vi "identify region.vi"(3 "index":u8=1, 4 "points":cluster{"x":i16, "y":i16}[](array[cluster]), 5 "location":cluster{"x":i16, "y":i16}, 6 "8-bit pixmap":u8[][](array[numeric])) -> (0 "distance":dbl, 2 "direction":dbl)   [LabVIEW 2009]
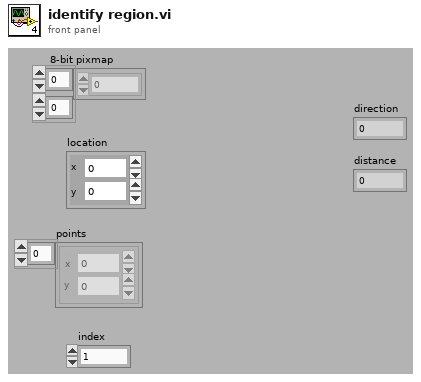
[diagram p1: front panel]
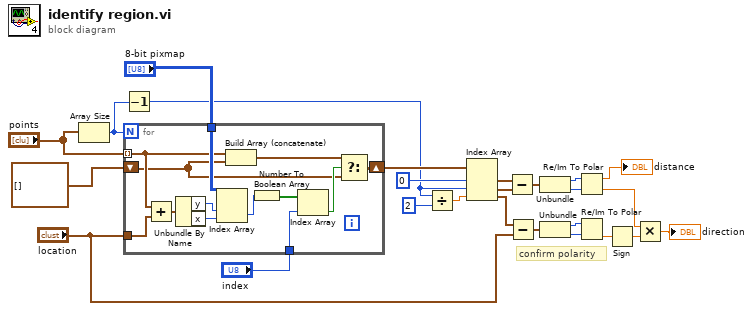
[diagram p0: block diagram]
diagram:
  # "confirm polarity"
  n1 = Array Size(array="points") -> (size(s)=w18:i32)
  n2 = Decrement(x=w18) -> (x-1=w12:i32)
  n3 = for {
    N: w18 -> [_]
    tunnel: "points" -> [w28] mode=indexing
    tunnel: "8-bit pixmap" -> [w38]
    shift-right: [w31] -> w19
    shift-left: cluster{"x":i16, "y":i16}[] [] ("points along perimeter") -> [w27]
    tunnel: "index" -> [w29]
    tunnel: "location" -> [w26]
    n4 = Add(x=w28, y=w26) -> (x+y=w34:cluster{"x":i16, "y":i16})
    n5 = Unbundle By Name(w34) -> ("y"=w32:i16, "x"=w33:i16)
    n6 = Index Array(array=w38, index (row)=w32, index (col)=w33) -> (element=w35:u8)
    n7 = Build Array (concatenate)(w28, w27) -> (w36:cluster{"x":i16, "y":i16}[])
    n8 = Number To Boolean Array(number=w35) -> (Boolean array=w37:bool[])
    n9 = Index Array(array=w37, index=w29) -> (element=w30:bool)
    n10 = Select(t=w36, s=w30, f=w27) -> (s? t:f=w31:cluster{"x":i16, "y":i16}[])
  }
  n11 = Divide(x=w12, y=2) -> (x/y=w10:dbl)
  n12 = Index Array(array=w19, index #1=0 ("index"), index #2=w12, index #3=w10) -> (element #1=w15:cluster{"x":i16, "y":i16}, element #2=w14:cluster{"x":i16, "y":i16}, element #3=w9:cluster{"x":i16, "y":i16})
  n13 = Subtract(x=w15, y=w14) -> (x-y=w22:cluster{"x":i16, "y":i16})
  n14 = Subtract(x=w9, y="location") -> (x-y=w5:cluster{"x":i16, "y":i16})
  n15 = Unbundle(w22) -> ("x"=w21:i16, "y"=w20:i16)
  n16 = Unbundle(w5) -> ("x"=w7:i16, "y"=w6:i16)
  n17 = Re/Im To Polar(2:w20, 3:w21) -> (0:w2:dbl, 1:→"distance":dbl)
  n18 = Re/Im To Polar(2:w6, 3:w7) -> (0:w4:dbl)  [unwired: 1 out]
  n19 = Sign(1:w4) -> (0:w3:dbl)
  n20 = Multiply(x=w2, y=w3) -> (x*y=→"direction":dbl)
